vi "Read_BT_Pkt.vi"(8 "error in":errorcluster, 11 "connection ID in":refnum<k31>) -> (0 "error out":errorcluster, 1 "Packet OK?":bool, 2 "Data":string, 3 "connection ID out":refnum<k31>)   [LabVIEW 2016]
panel:
  in  "bytes to read":i32=28
  out "packet_length":string
  in  "mode (standard)":T1(ring)
  out "sync_2":string
  out "sync_1":string
  out "Sync_1":i32
  out "Packet Size":u16
  out "Sync OK?":bool
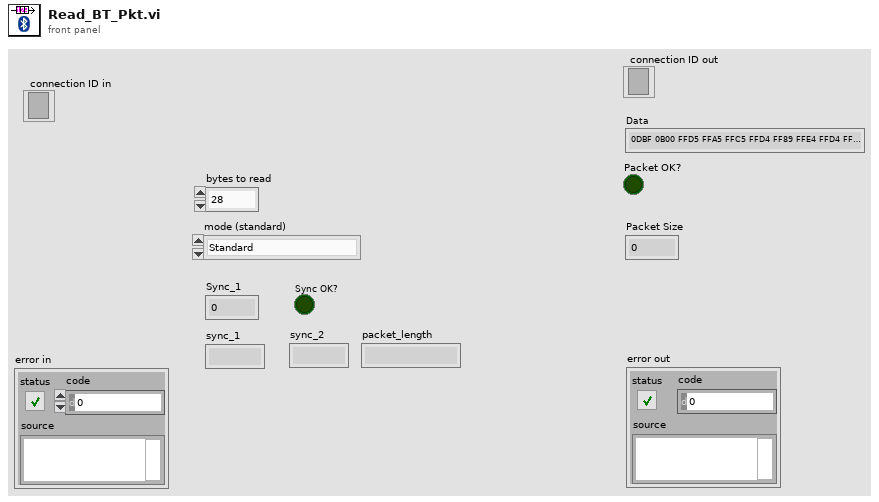
[diagram p1: front panel]
types:
  T1 = enum16{"Standard", "Buffered", "CRLF", "Immediate"}
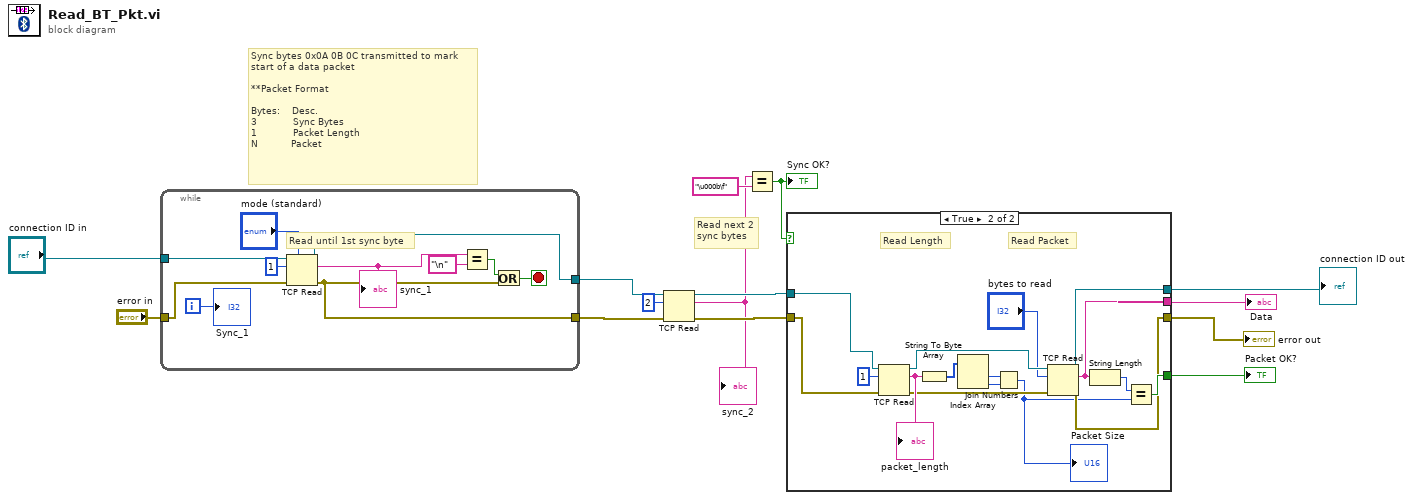
[diagram p0: block diagram]
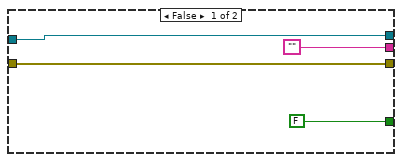
[diagram p2: hidden frame]
diagram:
  # "Sync bytes 0x0A 0B 0C transmitted to mark\nstart of a data packet\n\n**Packet Format\n\nBytes:    Desc.\n3            Sync Bytes\n1            Packet Length\nN           Packet"
  # "Read next 2\nsync bytes"
  n1 = while {
    tunnel: "connection ID in" -> [w19]
    tunnel: [w22] -> w7
    tunnel: [w20] -> w5
    tunnel: "error in" -> [w17]
    i -> [w18]
    stop <- w24 stop-if-true
    # "Read until 1st sync byte"
    n2 = TCP Read(connection ID=w19, bytes to read=1, error in (no error)=w17, 7:"mode (standard)") -> (connection ID out=w22:refnum<k31>, data out=w21:string, error out=w20:errorcluster)  [unwired: 1 in]
    "sync_1" <- w21
    n3 = Equal?(x=w21, y="\n") -> (x = y?=w23:bool)
    n4 = Or(x=w23, y=w20) -> (x .or. y?=w24:bool)
    "Sync_1" <- w18
  }
  n5 = TCP Read(connection ID=w7, bytes to read=2, error in (no error)=w5) -> (connection ID out=w6:refnum<k31>, data out=w3:string, error out=w4:errorcluster)  [unwired: 2 in]
  "sync_2" <- w3
  n6 = Equal?(x=w3, y="\u000b\f") -> (x = y?=w13:bool)
  "Sync OK?" <- w13
  n7 = case shown="True" w13 {
    tunnel: w6 -> [w29 w43]
    tunnel: w4 -> [w28 w42]
    tunnel: [w29 w37] -> w2
    tunnel: [w28 w38] -> w10
    tunnel: ["" w36] -> w11
    tunnel: [FALSE w44] -> w9
    frame False {
    }
    frame True {
      # "Read Length"
      # "Read Packet"
      n8 = TCP Read(connection ID=w43, bytes to read=1, error in (no error)=w42) -> (connection ID out=w40:refnum<k31>, data out=w41:string, error out=w39:errorcluster)  [unwired: 2 in]
      "packet_length" <- w41
      n9 = String To Byte Array(string=w41) -> (unsigned byte array=w45:u8[])
      n10 = Index Array(array=w45) -> (element #1=w31:u8, element #2=w30:u8)  [unwired: 2 in]
      n11 = Join Numbers(hi=w31, lo=w30) -> ((hi.lo)=w34:u16)
      "Packet Size" <- w34
      n12 = TCP Read(connection ID=w40, bytes to read="bytes to read", error in (no error)=w39) -> (connection ID out=w37:refnum<k31>, data out=w36:string, error out=w38:errorcluster)  [unwired: 2 in]
      n13 = String Length(string=w36) -> (length=w35:i32)
      n14 = Equal?(x=w35, y=w34) -> (x = y?=w44:bool)
    }
  }
  "error out" <- w10
  "Data" <- w11
  "Packet OK?" <- w9
  "connection ID out" <- w2
